vi "data_make_onehot.vi"() -> ()   [LabVIEW 2016]
uses:
  <vilib>/Utility/file.llb/Write Delimited Spreadsheet (DBL).vi
  <vilib>/Utility/file.llb/Read Delimited Spreadsheet (DBL).vi
panel:
  out "배열":dbl[][](array[numeric])
  in  "부분배열 2":dbl[](array[numeric])
  out "부분배열":dbl[](array[numeric])
  in  "비활성화된 인덱스 (열)":i32
  in  "all rows 2":dbl[][](array[numeric]) caption="모든 행"
  out "all rows":dbl[][](array[numeric]) caption="모든 행"
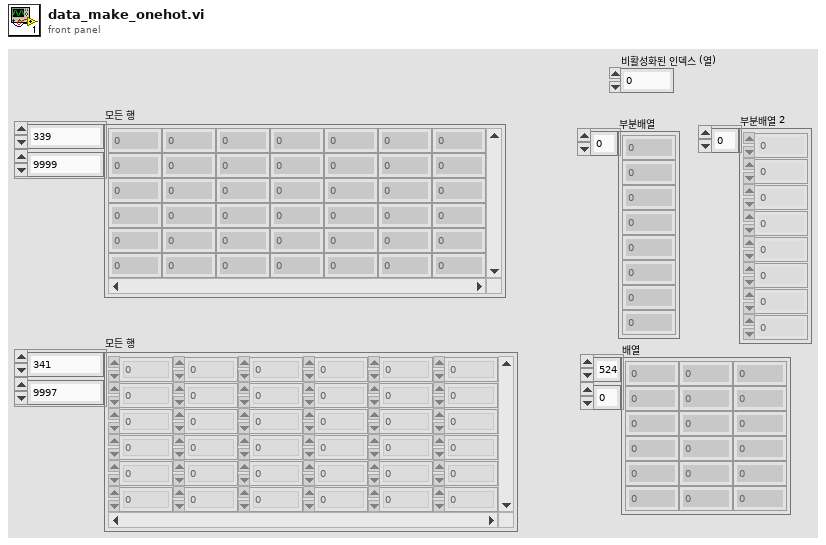
[diagram p1: front panel]
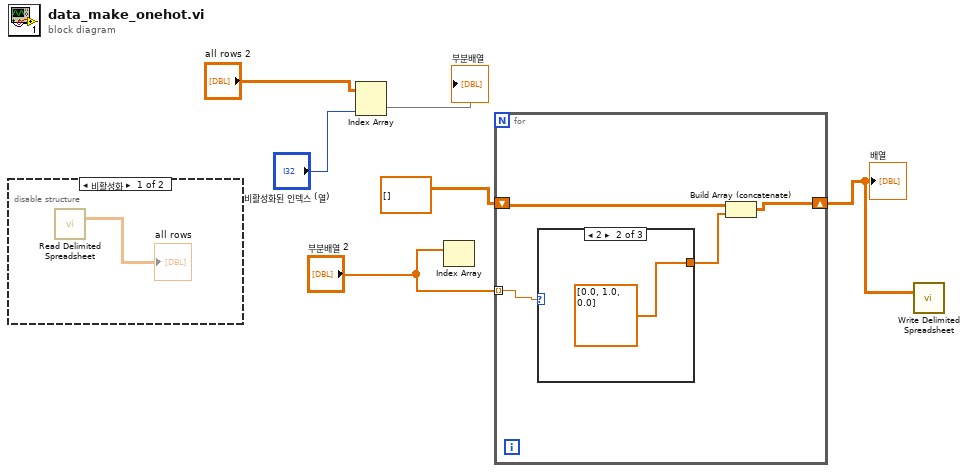
[diagram p0: block diagram]
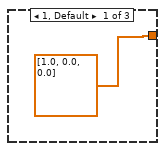
[diagram p2: hidden frame]
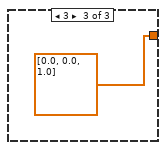
[diagram p3: hidden frame]
diagram:
  n1 = disable-structure shown="비활성화" {
    frame Disabled {
      n2 = call-poly <vilib>:"Read Delimited Spreadsheet.vi"() -> ("all rows"=→"all rows":dbl[][])  [unwired: 10 in, 5 out]
    }
    frame Enabled {
    }
  }
  n3 = Index Array(array="all rows 2", index (col)="비활성화된 인덱스 (열)") -> (element=→"부분배열":dbl[])  [unwired: 1 in]
  n4 = Index Array(array="부분배열 2") -> ()  [unwired: 1 in, 1 out]
  n5 = for {
    tunnel: "부분배열 2" -> [w10] mode=indexing
    shift-right: [w11] -> w1
    shift-left: dbl[][] [] -> [w8]
    n6 = case shown="2" w10 {
      tunnel: [dbl[] [1.0, 0.0, 0.0] dbl[] [0.0, 1.0, 0.0] dbl[] [0.0, 0.0, 1.0]] -> w9
      frame 1, Default {
      }
      frame 2 {
      }
      frame 3 {
      }
    }
    n7 = Build Array (concatenate)(w8, w9) -> (w11:dbl[][])
  }
  "배열" <- w1
  n8 = call-poly <vilib>:"Write Delimited Spreadsheet.vi"("2D data"=w1) -> ()  [unwired: 13 in, 2 out]
